vi "SoundSensorStart.vi"(0 "Device Info":T1={"Serial Number"=-1, "Channel"=0, "Port"=0}, 1 "Data Interval":i32=-1, 2 "Change Trigger":dbl, 5 "SPL Range":i32(ring)=1 items=["SPL_RANGE_102dB"=1, "SPL_RANGE_82dB"=2], 11 "error in (no error)":errorcluster, 12 "Connection":u16(ring) items=["No Preference", "Remote", "Local"], 13 "Timeout (mSec)":i32=5000) -> (4 "Phidget ID":u64, 6 "Serial Number Return":i32, 10 "Attached?":bool, 15 "error out":errorcluster)   [LabVIEW 2012, in "Phidget Sound Sensor.lvlib"]
doc: "${SoundSensor:StartHeader}"
uses:
  <instrlib>/Phidgets/Phidget Sound Sensor/Phidget Sound Sensor.lvlib
  <instrlib>/Phidgets/Phidget Common/Phidget Common.lvlib
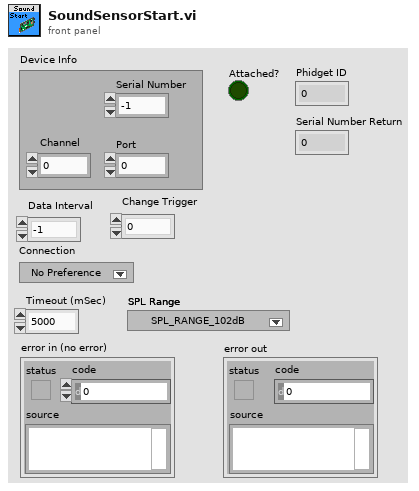
[diagram p1: front panel]
types:
  T1 = cluster{"Serial Number":i32, "Channel":i32, "Port":i32}
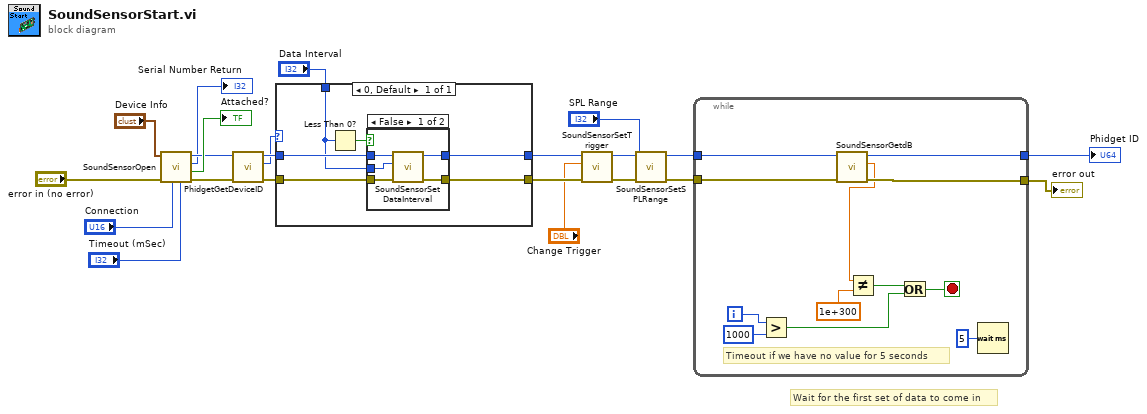
[diagram p0: block diagram]
diagram:
  # "Wait for the first set of data to come in"
  n1 = call <instrlib>:"SoundSensorOpen.vi"("Timeout (mSec)"="Timeout (mSec)", "Connection"="Connection", "error in"="error in (no error)", "Device Info"="Device Info") -> ("error out"=w19:errorcluster, "Attached?"=→"Attached?":bool, "Serial Number Return"=→"Serial Number Return":i32, "Phidget ID"=w18:u64)  [unwired: 4 in]
  n2 = call <instrlib>:"PhidgetGetDeviceID.vi"("error in (no error)"=w19, "Device In"=w18) -> ("error out"=w16:errorcluster, "Devie IDs"=w15:u32, "Device Out"=w17:u64)  [unwired: 6 in]
  n3 = case shown="0, Default" w15 {
    tunnel: w16 -> [w27]
    tunnel: [w23] -> w11
    tunnel: w17 -> [w26]
    tunnel: [w24] -> w12
    tunnel: "Data Interval" -> [w25]
    frame 0, Default {
      n4 = Less Than 0?(x=w25) -> (x < 0?=w28:bool)
      n5 = case shown="False" w28 {
        tunnel: w26 -> [w33 w35]
        tunnel: w27 -> [w32 w34]
        tunnel: [w30 w35] -> w24
        tunnel: [w31 w34] -> w23
        tunnel: w25 -> [w29 _]
        frame False {
          n6 = call <instrlib>:"SoundSensorSetDataInterval.vi"("error in (no error)"=w32, "Interval"=w29, "Device In"=w33) -> ("error out"=w31:errorcluster, "Device Out"=w30:u64)  [unwired: 6 in]
        }
        frame True {
        }
      }
    }
  }
  n7 = call <instrlib>:"SoundSensorSetTrigger.vi"("error in (no error)"=w11, "Trigger"="Change Trigger", "Device In"=w12) -> ("error out"=w3:errorcluster, "Device Out"=w5:u64)  [unwired: 6 in]
  n8 = call <instrlib>:"SoundSensorSetSPLRange.vi"("error in (no error)"=w3, "SPL Range"="SPL Range", "Device In"=w5) -> ("error out"=w2:errorcluster, "Device Out"=w4:u64)  [unwired: 6 in]
  n9 = while {
    tunnel: w4 -> [w45]
    tunnel: w2 -> [w44]
    tunnel: [w42] -> w14
    tunnel: [w43] -> w21
    i -> [w40]
    stop <- w37 stop-if-true
    # "Timeout if we have no value for 5 seconds"
    n10 = Greater?(x=w40, y=1000) -> (0:w38:bool)
    n11 = call <instrlib>:"SoundSensorGetdB.vi"("error in (no error)"=w44, "Device In"=w45) -> ("error out"=w43:errorcluster, "dB"=w36:dbl, "Device Out"=w42:u64)  [unwired: 6 in]
    n12 = Not Equal?(x=w36, y=1e+300) -> (x != y?=w39:bool)
    n13 = Or(x=w39, y=w38) -> (x .or. y?=w37:bool)
    n14 = Wait (ms)(milliseconds to wait=u32 5) -> ()  [unwired: 1 out]
  }
  "error out" <- w21
  "Phidget ID" <- w14
